vi "In-Line-Pressure.vi"(2 "Zero Pressure\n(F = leave as is)":bool=TRUE, 3 "In-Line Pressure Slope":dbl=47.84 format="%.2f", 4 "In-Line Pressure Offset":dbl=40.0 format="%.2f") -> (1 "Pressure":dbl=0.003808000000006473 format="%.2f")   [LabVIEW 2016]
uses:
  Kpro Globals.vi
panel:
  out "Voltage":dbl=0.8362 format="%.3f"
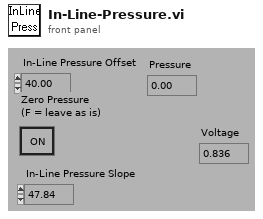
[diagram p1: front panel]
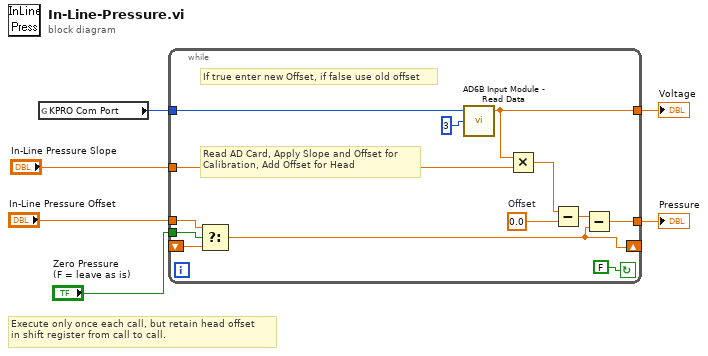
[diagram p0: block diagram]
diagram:
  # "Execute only once each call, but retain head offset \nin shift register from call to call."
  n1 = global read "Kpro Globals.vi" "KPRO Com Port"() -> (w3:i32)
  n2 = while {
    tunnel: "Zero Pressure\n(F = leave as is)" -> [w14]
    tunnel: "In-Line Pressure Offset" -> [w15]
    shift-left: _ -> [w16]
    shift-right: [w10] -> _
    tunnel: [w13] -> w6
    tunnel: w3 -> [w9]
    tunnel: "In-Line Pressure Slope" -> [w7]
    tunnel: [w8] -> w1
    stop <- FALSE continue-if-true
    w17 = 0.0  # Offset
    # "Read AD Card, Apply Slope and Offset for\nCalibration, Add Offset for Head"
    # "If true enter new Offset, if false use old offset"
    n3 = Select(t=w15, s=w14, f=w16) -> (s? t:f=w10:dbl)
    n4 = call "AD6B Input Module - Read Data.VI"("address (0 to 255)"=3, "port number (1:com2)"=w9) -> ("scaled data"=w8:dbl)  [unwired: 1 in, 2 out]
    n5 = Multiply(x=w8, y=w7) -> (x*y=w18:dbl)
    n6 = Subtract(x=w18, y=w17) -> (x-y=w11:dbl)
    n7 = Subtract(x=w11, y=w10) -> (x-y=w13:dbl)
  }
  "Pressure" <- w6
  "Voltage" <- w1
